vi "Set Elements Owner.vi"(8 "error in (no error)":errorcluster, 11 "Config Manager in":refnum<class "Config Manager.lvclass">) -> (0 "error out":errorcluster, 3 "Config Manager out":refnum<class "Config Manager.lvclass">)   [LabVIEW 2020, in "CDM-Config.lvlib" / "Config Manager.lvclass"]
uses:
  Config Manager.lvclass
  Config Manager.lvclass/Config Manager.ctl
  Config Element/Config Element.lvclass
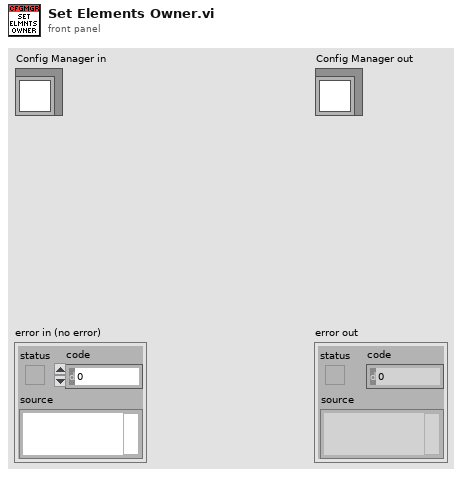
[diagram p1: front panel]
types:
  T1 = typedef "CDM-Config.lvlib/Config Manager.lvclass/Ref Data.ctl" = cluster{"Elements":refnum<class "Config Element.lvclass">[], "Hierarchy Map":map{string[], i32}, "Element Map":map{refnum<class "Config Element.lvclass">, i32}}
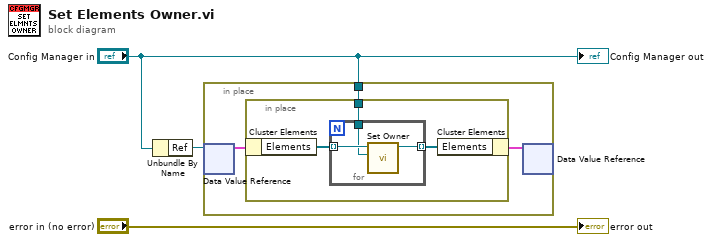
[diagram p0: block diagram]
diagram:
  n1 = Unbundle By Name("Config Manager in") -> ("Ref"=w2:refnum<data-value>)
  n2 = in-place {
    in-place-border: "Config Manager in" -> [w4]
    n3 = in-place-dvr #1(w2) -> (w6:T1)  [unwired: 1 out]
    n4 = in-place {
      in-place-border: w4 -> [w8]
      n5 = in-place-cluster #2(w6) -> ("Elements"=w9:refnum<class "Config Element.lvclass">[])
      n6 = for {
        tunnel: w9 -> [w12] mode=indexing
        tunnel: w8 -> [w11]
        tunnel: [w10] -> w7 mode=indexing
        n7 = call "Set Owner.vi"("Owner"=w11, "Config Element in"=w12) -> ("Config Element out"=w10:refnum<class "Config Element.lvclass">)  [unwired: 8 in, 1 out]
      }
      n8 = in-place-cluster #2("Elements"=w7) -> (w5:T1)
    }
    n9 = in-place-dvr #1(w5) -> ()  [unwired: 2 out]
  }
  "error out" <- "error in (no error)"
  "Config Manager out" <- "Config Manager in"
